vi "Set Configuration Data.vi"(8 "error in (no error)":errorcluster, 10 "configuration data":T1, 11 "configuration session in":refnum<class "Configuration Session.lvclass">) -> (0 "error out":errorcluster, 3 "configuration session out":refnum<class "Configuration Session.lvclass">)   [LabVIEW 2021, in "DSF Core.lvlib" / "Configuration Session.lvclass"]
doc: "Reads a value associated with a key in a specified section from the configuration data identified by <B>dsf refnum</B>. If the key does not exist, the VI returns the default value. This VI supports multibyte characters in strings. Wire data to the <B>default value</B> input to determine the polymorphic instance to use or manually select the instance."
uses:
  Configuration Session.lvclass
  Typedefs/DSF Engine Framework Configuration.ctl
  Typedefs/DSF Engine Plugin Configuration.ctl
  Typedefs/Core Plugin Configuration.ctl
  Typedefs/DSF Timing Info.ctl
  Typedefs/DSF Settings Info.ctl
  Typedefs/DSF Engine Plugin Thread Configuration.ctl
  Typedefs/Core Thread Configuration.ctl
  Typedefs/DSF Engine Transfer Group Configuration.ctl
  Typedefs/Core Group Configuration.ctl
  Typedefs/DSF Direction.ctl
  Typedefs/DSF Timeout Behavior.ctl
  Typedefs/DSF Engine Transfer Configuration.ctl
  Typedefs/Core Transfer Configuration.ctl
  Typedefs/DSF Engine Channel Configuration.ctl
  Typedefs/Core Channel Configuration.ctl
  Typedefs/DSF Data Type.ctl
  Configuration Session.lvclass/Configuration Session.ctl
  DSF Core.lvlib
  Configuration/Core/Channel/Channel Configuration.lvclass
  Configuration/Core/Transfer/Transfer Configuration.lvclass
  Configuration/Core/Group/Group Configuration.lvclass
  Configuration/Core/Thread/Thread Configuration.lvclass
  Configuration/Core/Plugin/Plugin Configuration.lvclass
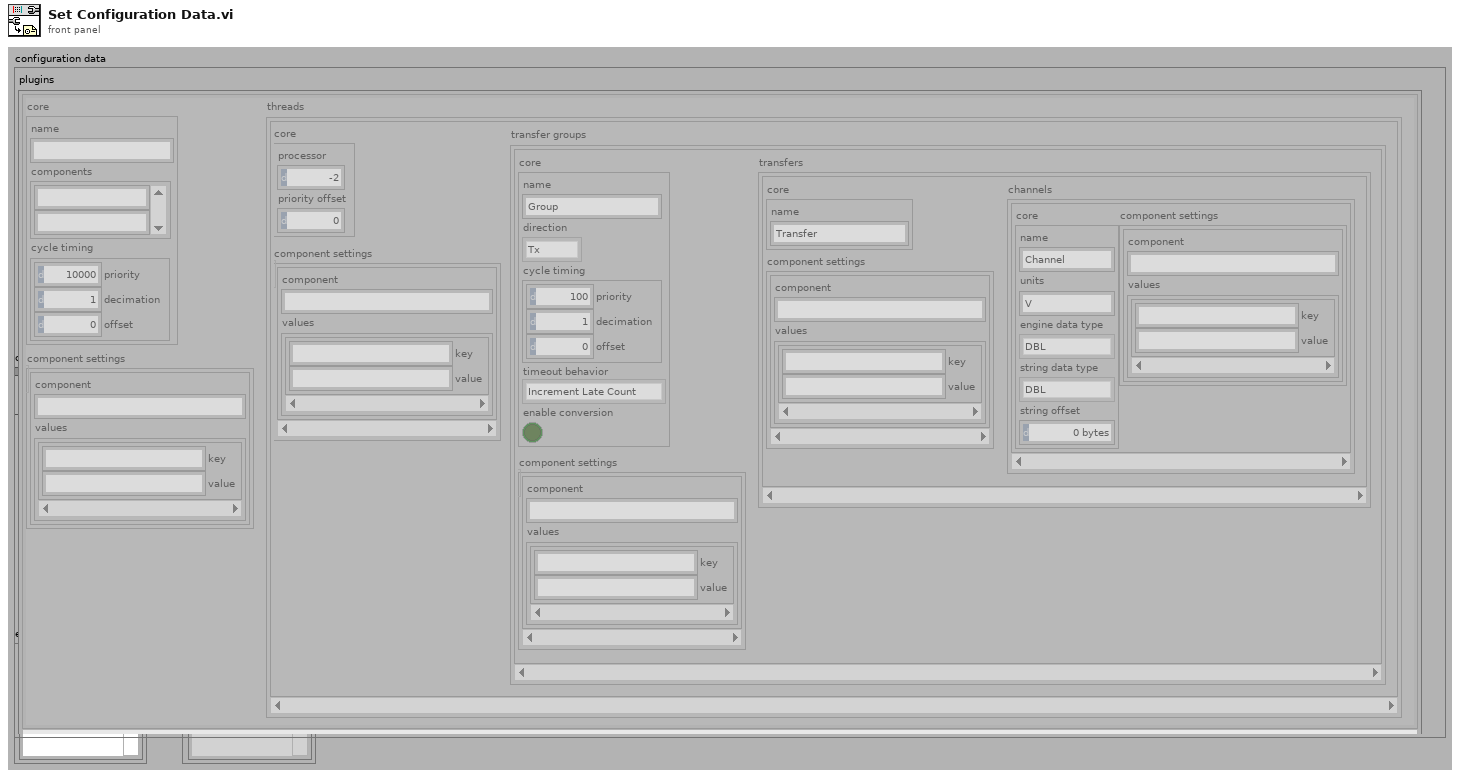
[diagram p1: front panel]
types:
  T1 = typedef "DSF Core.lvlib/DSF Engine Framework Configuration.ctl" = cluster{"plugins":T2[]}
  T2 = typedef "DSF Core.lvlib/DSF Engine Plugin Configuration.ctl" = cluster{"core":T3, "component settings":T5[], "threads":T6[]}
  T3 = typedef "DSF Core.lvlib/Plugin Configuration.lvclass/Core Plugin Configuration.ctl" = cluster{"name":string, "components":string[], "cycle timing":T4}
  T4 = typedef "DSF Core.lvlib/DSF Timing Info.ctl" = cluster{"priority":u64, "decimation":u64, "offset":u64}
  T5 = typedef "DSF Core.lvlib/DSF Settings Info.ctl" = cluster{"component":string, "values":cluster{"key":string, "value":string}[]}
  T6 = typedef "DSF Core.lvlib/DSF Engine Plugin Thread Configuration.ctl" = cluster{"core":T7, "component settings":T5[], "transfer groups":T8[]}
  T7 = typedef "DSF Core.lvlib/Thread Configuration.lvclass/Core Thread Configuration.ctl" = cluster{"processor":i32, "priority offset":i16}
  T8 = typedef "DSF Core.lvlib/DSF Engine Transfer Group Configuration.ctl" = cluster{"core":T9, "component settings":T5[], "transfers":T12[]}
  T9 = typedef "DSF Core.lvlib/Group Configuration.lvclass/Core Group Configuration.ctl" = cluster{"name":string, "direction":T10, "cycle timing":T4, "timeout behavior":T11, "enable conversion":bool}
  T10 = typedef "DSF Core.lvlib/DSF Direction.ctl" = enum8{"Tx", "Rx"}
  T11 = typedef "DSF Core.lvlib/DSF Timeout Behavior.ctl" = enum8{"Increment Late Count", "Throw Error"}
  T12 = typedef "DSF Core.lvlib/DSF Engine Transfer Configuration.ctl" = cluster{"core":T13, "component settings":T5[], "channels":T14[]}
  T13 = typedef "DSF Core.lvlib/Transfer Configuration.lvclass/Core Transfer Configuration.ctl" = cluster{"name":string}
  T14 = typedef "DSF Core.lvlib/DSF Engine Channel Configuration.ctl" = cluster{"core":T15, "component settings":T5[]}
  T15 = typedef "DSF Core.lvlib/Channel Configuration.lvclass/Core Channel Configuration.ctl" = cluster{"name":string, "units":string, "engine data type":T16, "string data type":T16, "string offset":u64}
  T16 = typedef "DSF Core.lvlib/DSF Data Type.ctl" = enum8{"Bool", "SGL", "DBL", "I8", "I16", "I32", "I64", "U8", "U16", "U32", "U64"}
  T17 = typedef "DSF Core.lvlib/Configuration Session.lvclass/DSF Config Data Ref.ctl" = refnum<data-value>
  T18 = typedef "DSF Core.lvlib/Configuration Session.lvclass/DSF Config Data.ctl" = cluster{"dsf configuration":T19, "path":path, "dirty":bool}
  T19 = typedef "DSF Core.lvlib/Configuration Session.lvclass/Internal DSF Configuration.ctl" = cluster{"dsfversion":T20, "version":T20, "plugins":T21[], "groups":T23[], "transfers":T25[], "channels":T27[], "settings":T29[], "framework configuration":T1, "configuration":refnum<class>}
  T20 = typedef "DSF Core.lvlib/DSF Version Info.ctl" = cluster{"major":u32, "minor":u32, "fix":u32, "build":string}
  T21 = typedef "DSF Core.lvlib/Configuration Session.lvclass/Internal DSF Plugin with ID.ctl" = cluster{"id":string, "values":T22}
  T22 = typedef "DSF Core.lvlib/Configuration Session.lvclass/Internal DSF Plugin Info.ctl" = cluster{"components":string[], "timing":T4, "group ids":string[], "settings id":string, "threads":T6[]}
  T23 = typedef "DSF Core.lvlib/Configuration Session.lvclass/Internal DSF Group with ID.ctl" = cluster{"id":string, "values":T24}
  T24 = typedef "DSF Core.lvlib/Configuration Session.lvclass/Internal DSF Group Info.ctl" = cluster{"direction":i32, "timing":T4, "transfer ids":string[], "settings id":string, "thread":i32, "timeout behavior":u8}
  T25 = typedef "DSF Core.lvlib/Configuration Session.lvclass/Internal DSF Transfer with ID.ctl" = cluster{"id":string, "values":T26}
  T26 = typedef "DSF Core.lvlib/Configuration Session.lvclass/Internal DSF Transfer Info.ctl" = cluster{"byte order":i32, "channel ids":string[], "settings id":string}
  T27 = typedef "DSF Core.lvlib/Configuration Session.lvclass/Internal DSF Channel with ID.ctl" = cluster{"id":string, "values":T28}
  T28 = typedef "DSF Core.lvlib/Configuration Session.lvclass/Internal DSF Channel Info.ctl" = cluster{"string buffer offset":u64, "string data type":i32, "engine data type":i32, "settings id":string, "units":string}
  T29 = typedef "DSF Core.lvlib/Configuration Session.lvclass/Internal DSF Settings with ID.ctl" = cluster{"id":string, "values":T30}
  T30 = typedef "DSF Core.lvlib/Configuration Session.lvclass/Internal DSF Settings Info.ctl" = cluster{"key":string, "value":string}[]
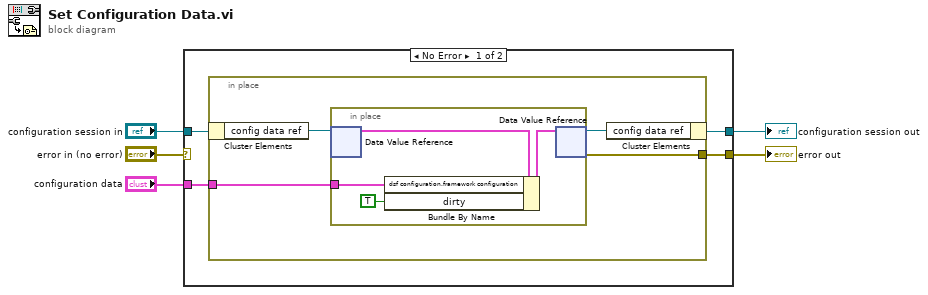
[diagram p0: block diagram]
diagram:
  n1 = case shown="No Error" "error in (no error)" {
    selector: "error in (no error)" -> [_ w19]
    tunnel: "configuration session in" -> [w7 w18]
    tunnel: [w8 w19] -> w4
    tunnel: "configuration data" -> [w9 _]
    tunnel: [w6 w18] -> w1
    frame No Error {
      n2 = in-place {
        in-place-border: w9 -> [w13]
        in-place-border: [w12] -> w8
        n3 = in-place-cluster #1(w7) -> ("config data ref"=w11:T17)
        n4 = in-place {
          in-place-border: w13 -> [w17]
          n5 = in-place-dvr #2(w11) -> (w16:T18)  [unwired: 1 out]
          n6 = Bundle By Name(cluster=w16, "dsf configuration.framework configuration"=w17, "dirty"=TRUE) -> (w15:T18)
          n7 = in-place-dvr #2(w15) -> (w10:T17, w12:errorcluster)
        }
        n8 = in-place-cluster #1("config data ref"=w10) -> (w6:refnum<class "Configuration Session.lvclass">)
      }
    }
    frame Error {
    }
  }
  "error out" <- w4
  "configuration session out" <- w1
